vi "Interpolate 1D.vi"(6 "ntimes":i32=1, 7 "method":i32(ring)=1 items=["nearest", "linear", "spline", "cubic Hermite", "Lagrange"], 8 "X is monotonic":bool, 9 "xi":dbl[](array[numeric]) format="%_6g", 10 "X":dbl[](array[numeric]) format="%_6g", 11 "Y":dbl[](array[numeric]) format="%_6g") -> (0 "error":i32, 2 "xi used":dbl[](array[numeric]) format="%_6g", 3 "yi":dbl[](array[numeric]) format="%_6g")   [LabVIEW 2017, in "NI_Gmath.lvlib"]
doc: "Performs one-dimensional interpolation using a selected method based on the lookup table defined by <B>X</B> and <B>Y</B>."
uses:
  NI_Gmath.lvlib
panel:
  # "Interpolate 1D"
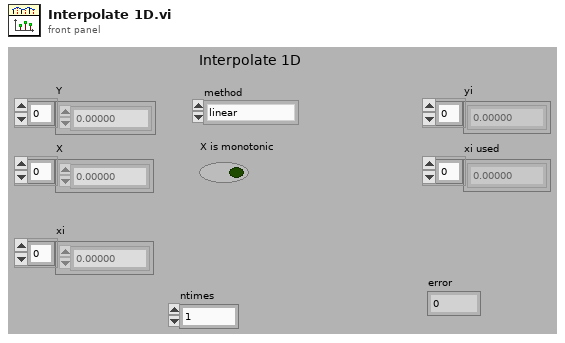
[diagram p1: front panel]
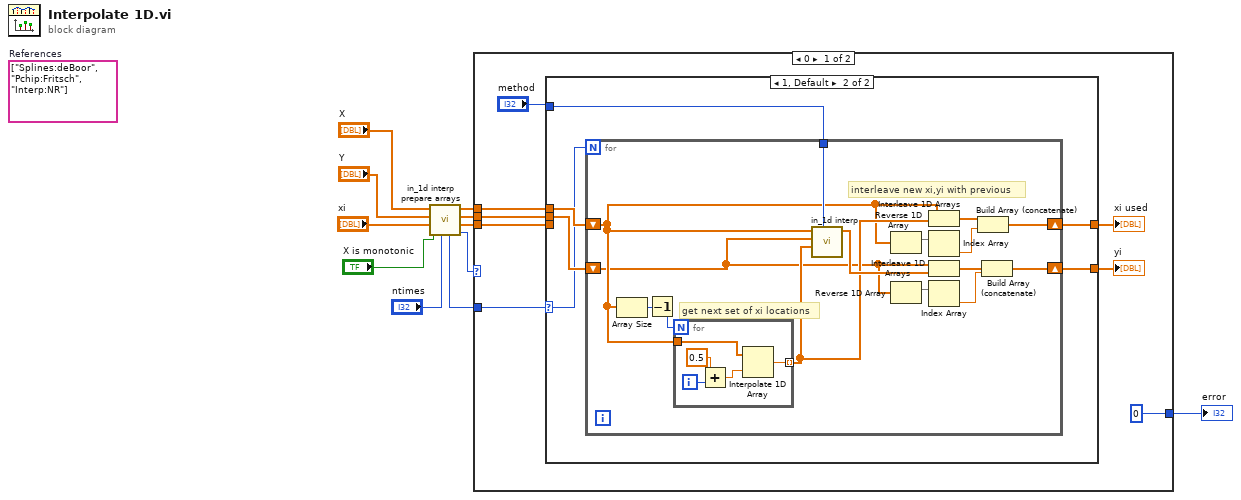
[diagram p0: block diagram]
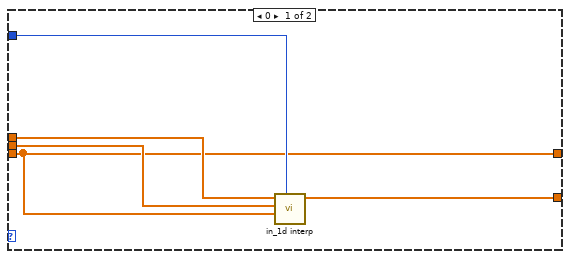
[diagram p2: hidden frame]
diagram:
  (unwired) string[] ["Splines:deBoor", "Pchip:Fritsch", "Interp:NR"]  # References
  n1 = call "in_1d interp prepare arrays.vi"("ntimes"="ntimes", "X is monotonic"="X is monotonic", "xi"="xi", "Y"="Y", "X"="X") -> ("error"=w2:i32, "xi-out"=w6:dbl[], "Y-out"=w7:dbl[], "X-out"=w8:dbl[], "ntimes remaining"=w4:i32)  [unwired: 2 in]
  n2 = case shown="0" w2 {
    selector: w2 -> [_ w51]
    tunnel: w8 -> [w19 _]
    tunnel: w7 -> [w18 _]
    tunnel: w6 -> [w17 _]
    tunnel: w4 -> [w13 _]
    tunnel: [0 ("error") w51] -> w3
    frame 0 {
      n3 = case shown="1, Default" w13 {
        selector: w13 -> [_ w25]
        tunnel: w19 -> [w24 w30]
        tunnel: w18 -> [w23 w27]
        tunnel: w17 -> [w20 _]
        tunnel: [w22 w28] -> w16
        tunnel: "method" -> [w21 w29]
        tunnel: [w20 w26] -> w14
        frame 0 {
          n4 = call "in_1d interp.vi"("method"=w21, "xi"=w20, "Y"=w23, "X"=w24) -> ("yi"=w22:dbl[])  [unwired: 6 in, 1 out]
        }
        frame 1, Default {
          n5 = for {
            N: w25 -> [_]
            tunnel: w29 -> [w45]
            shift-right: [w39] -> w26
            shift-left: w30 -> [w36]
            shift-right: [w37] -> w28
            shift-left: w27 -> [w31]
            # "get next set of xi locations"
            # "interleave new xi,yi with previous"
            n6 = Array Size(array=w36) -> (size(s)=w42:i32)
            n7 = Decrement(x=w42) -> (x-1=w41:i32)
            n8 = for {
              N: w41 -> [_]
              tunnel: [w50] -> w40 mode=indexing
              tunnel: w36 -> [w46]
              i -> [w48]
              n9 = Add(x=0.5, y=w48) -> (x+y=w47:dbl)
              n10 = Interpolate 1D Array(1:w47, 2:w46) -> (0:w50:dbl)
            }
            n11 = call "in_1d interp.vi"("method"=w45, "xi"=w40, "Y"=w31, "X"=w36) -> ("yi"=w44:dbl[])  [unwired: 6 in, 1 out]
            n12 = Reverse 1D Array(array=w36) -> (reversed array=w35:dbl[])
            n13 = Reverse 1D Array(array=w31) -> (reversed array=w33:dbl[])
            n14 = Interleave 1D Arrays(w36, w40) -> (w43:dbl[])
            n15 = Index Array(array=w35) -> (element=w34:dbl)  [unwired: 1 in]
            n16 = Interleave 1D Arrays(w31, w44) -> (w38:dbl[])
            n17 = Index Array(array=w33) -> (element=w32:dbl)  [unwired: 1 in]
            n18 = Build Array (concatenate)(w43, w34) -> (w39:dbl[])
            n19 = Build Array (concatenate)(w38, w32) -> (w37:dbl[])
          }
        }
      }
      "yi" <- w16
      "xi used" <- w14
    }
    frame Default {
    }
  }
  "error" <- w3
